vi "ErrorLatch.vi"(1 "Trigger":bool) -> (0 "Latched":bool)   [LabVIEW 2019]
doc: "This VI will latch an error flag until cleared or suppressed (overriden). This VI is designed for integration with global variables to read the error clear and override signals."
panel:
  in  "Clear Errors[PLACEHOLDER]":bool
  in  "Master Safety Override [PLACEHOLDER]":bool
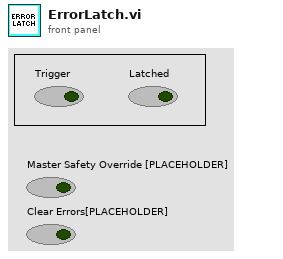
[diagram p1: front panel]
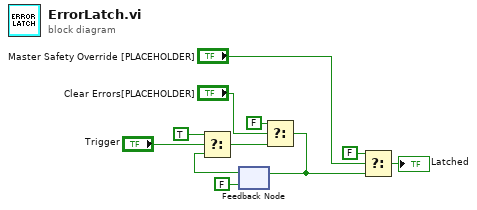
[diagram p0: block diagram]
diagram:
  n1 = feedback #1(FALSE) -> (w10:bool)
  n2 = Select(t=TRUE, s="Trigger", f=w10) -> (s? t:f=w7:bool)
  n3 = Select(t=FALSE, s="Clear Errors[PLACEHOLDER]", f=w7) -> (s? t:f=w5:bool)
  n4 = feedback-in #1(w5) -> ()
  n5 = Select(t=FALSE, s="Master Safety Override [PLACEHOLDER]", f=w5) -> (s? t:f=→"Latched":bool)
